vi "Format LUT String.vi"(11 "Input String":string) -> (3 "Output String":string)   [LabVIEW 2018, in "Assert API Components.lvlib" / "Process Monitor.lvlib"]
uses:
  Process Monitor.lvlib
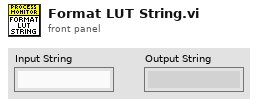
[diagram p1: front panel]
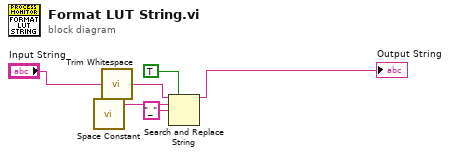
[diagram p0: block diagram]
diagram:
  n1 = call <vilib>:"Space Constant.vi"() -> ("String"=w3:string)
  n2 = call <vilib>:"Trim Whitespace.vi"("string"="Input String") -> ("trimmed string"=w2:string)  [unwired: 1 in]
  n3 = Search and Replace String(replace all?=TRUE ("replace all? (F)"), input string=w2, search string=w3, replace string="_" ("replace string (\"\")")) -> (result string=→"Output String":string)  [unwired: 4 in, 3 out]
